vi "SR430.destructor.vi"(0 "i ref in":refnum<vi>, 5 "error in (no error)":errorcluster) -> (19 "error out":errorcluster)   [LabVIEW 2014, in "SR430.lvlib"]
doc: "This is the destructor of a class.\n\nLicense Agreement for this software:\n\nCopyright (C)\nGesellschaft für Schwerionenforschung, GSI\nPlanckstr. 1\n64291 Darmstadt\nGermany\n\nContact: D.Beck@gsi.de \n\nThis program is free software; you can redistribute it and/or modify it under the terms of the \nGNU General Public License as published by the Free Software Foundation; either version 2 of \nthe license, or (at your option) any later version.\n\nThis program is distributed in the hope that it will be useful, but WITHOUT ANY WARRANTY; \nwithout even the implied warranty of MERCHANTABILITY or FITNESS FOR A PARTICULAR PURPOSE. See the GNU General License for more details (http://www.gnu.org).\n\nGesellschaft für Schwerionenforschung, GSI\nPlanckstr. 1, 64291 Darmstadt, Germany\nFor all questions and ideas contact: M.Richter@gsi.de, H.Brand@gsi.de or D.Beck@gsi.de.\nLast update: 16-JUN-2004"
uses:
  SR430.lvlib
  CSinstr.lib/Sr430/SR430Driver.lvlib
  CSCore/CSApplicationBaseClasses/MCSBase/MCSBase.lvlib
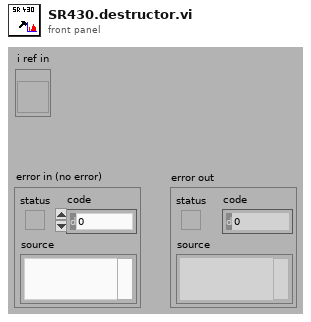
[diagram p1: front panel]
types:
  T1 = typedef "SR430.lvlib/SR430.i attribute.ctl" = cluster{"initialized":bool, "SR430 VISA Cluster":T2}
  T2 = typedef "SR430Driver.lvlib/SR430_VISA Control.ctl" = cluster{"VISA resource name":refnum<visa-resource-name>}
  T3 = enum16{"SetAttribute", "GetAttribute", "CreateAttribute", "DestroyAttribute", "DestroyAllAtributes"}
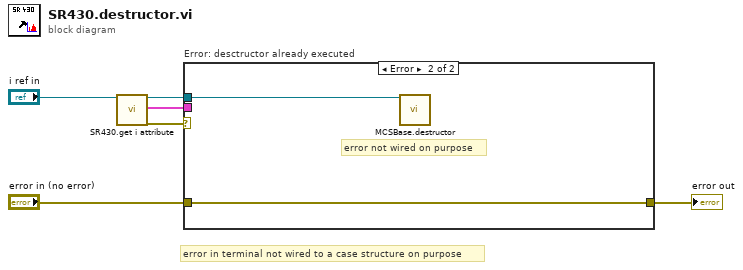
[diagram p0: block diagram]
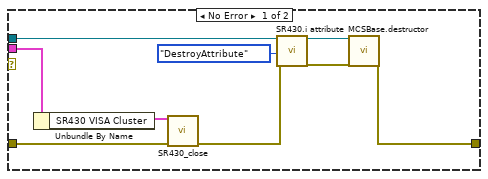
[diagram p2: hidden frame]
diagram:
  # "error in terminal not wired to a case structure on purpose"
  n1 = call "SR430.get i attribute.vi"("i ref in"="i ref in") -> ("i ref out"=w3:refnum<vi>, "i attribute"=w1:T1, "error out"=w2:errorcluster)  [unwired: 16 in]
  n2 = case "Error: desctructor already executed" shown="Error" w2 {
    tunnel: [w12 w17] -> w6
    tunnel: "error in (no error)" -> [w8 w17]
    tunnel: w3 -> [w11 w16]
    tunnel: w1 -> [w10 _]
    frame No Error {
      n3 = Unbundle By Name(w10) -> ("SR430 VISA Cluster"=w9:T2)
      n4 = call "SR430_close.vi"("SR430 VISA Cluster"=w9, "error in (no error)"=w8) -> ("error out"=w7:errorcluster)  [unwired: 13 in]
      n5 = call "SR430.i attribute.vi"("VI Refnum"=w11, "Action"=T3."DestroyAttribute", "error in (no error)"=w7) -> ("VI Refnum out"=w14:refnum<vi>, "error out"=w13:errorcluster)  [unwired: 14 in, 1 out]
      n6 = call "MCSBase.destructor.vi"("i ref in"=w14, "error in (no error)"=w13) -> ("error out"=w12:errorcluster)  [unwired: 17 in]
    }
    frame Error {
      # "error not wired on purpose"
      n7 = call "MCSBase.destructor.vi"("i ref in"=w16) -> ()  [unwired: 18 in, 1 out]
    }
  }
  "error out" <- w6
